vi "Collide_flappy.vi"(6 "Test":bool, 7 "obs_a?":bool, 8 "error in":errorcluster, 9 "Obs D_in":refnum<vi>[](array[refnum]), 10 "Obs U_in":refnum<vi>[](array[refnum]), 11 "ball in":refnum<vi>) -> (0 "error Out":errorcluster, 2 "bump":bool)   [LabVIEW 2014]
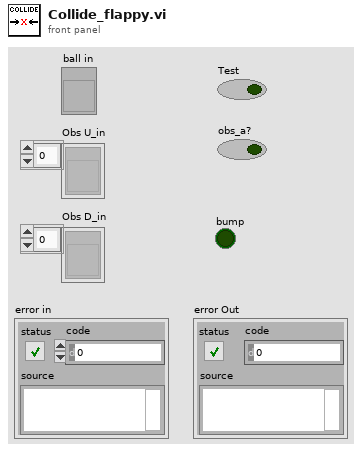
[diagram p1: front panel]
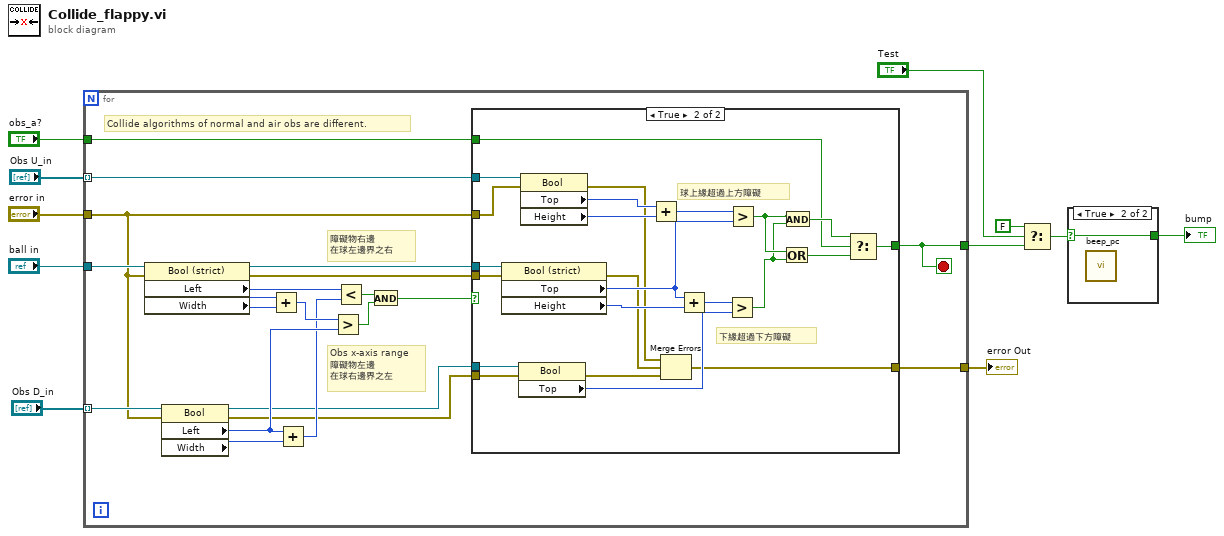
[diagram p0: block diagram]
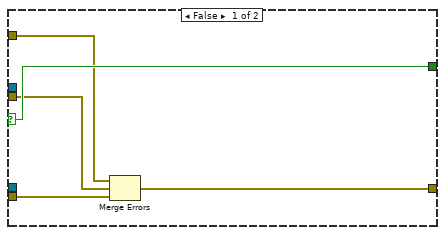
[diagram p3: hidden frame]
diagram:
  n1 = for {
    tunnel: "Obs U_in" -> [w22] mode=indexing
    tunnel: "ball in" -> [w21]
    tunnel: "Obs D_in" -> [w20] mode=indexing
    tunnel: "error in" -> [w15]
    tunnel: [w13] -> w3
    tunnel: [w14] -> w9
    tunnel: "obs_a?" -> [w12]
    stop <- w13 stop-if-true
    # "Collide algorithms of normal and air obs are different."
    # "障礙物右邊\n在球左邊界之右"
    # "Obs x-axis range\n障礙物左邊\n在球右邊界之左"
    n2 = property on="Property Node" class="Bool (strict)"(reference=w21, error in=w15) -> (reference out=w18:refnum<vi>, error out=w17:errorcluster, "Left"=w25:i32, "Width"=w26:u32)
    n3 = property on="Property Node" class="Bool"(reference=w20, error in=w15) -> (reference out=w19:refnum<vi>, error out=w16:errorcluster, "Left"=w28:i32, "Width"=w23:u32)
    n4 = Add(x=w25, y=w26) -> (x+y=w27:u32)
    n5 = Add(x=w28, y=w23) -> (x+y=w24:u32)
    n6 = Greater?(x=w27, y=w28) -> (0:w30:bool)
    n7 = Less?(x=w25, y=w24) -> (x < y?=w29:bool)
    n8 = And(x=w29, y=w30) -> (x .and. y?=w31:bool)
    n9 = case shown="True" w31 {
      selector: w31 -> [w36 _]
      tunnel: [w36 w41] -> w13
      tunnel: w22 -> [_ w54]
      tunnel: w18 -> [_ w53]
      tunnel: w19 -> [_ w52]
      tunnel: w17 -> [w33 w51]
      tunnel: w16 -> [w35 w50]
      tunnel: w15 -> [w32 w49]
      tunnel: [w34 w43] -> w14
      tunnel: w12 -> [_ w39]
      frame False {
        n10 = Merge Errors(w32, w33, w35) -> (w34:errorcluster)
      }
      frame True {
        # "球上緣超過上方障礙"
        # "下緣超過下方障礙"
        n11 = property on="Property Node" class="Bool (strict)"(reference=w53, error in=w51) -> (error out=w46:errorcluster, "Top"=w48:i32, "Height"=w57:u32)  [unwired: 1 out]
        n12 = property on="Property Node" class="Bool"(reference=w52, error in=w50) -> (error out=w45:errorcluster, "Top"=w55:i32)  [unwired: 1 out]
        n13 = property on="Property Node" class="Bool"(reference=w54, error in=w49) -> (error out=w44:errorcluster, "Top"=w58:i32, "Height"=w59:u32)  [unwired: 1 out]
        n14 = Add(x=w58, y=w59) -> (x+y=w47:u32)
        n15 = Merge Errors(w44, w46, w45) -> (w43:errorcluster)
        n16 = Add(x=w48, y=w57) -> (x+y=w56:u32)
        n17 = Greater?(x=w56, y=w55) -> (0:w37:bool)
        n18 = Greater?(x=w47, y=w48) -> (0:w38:bool)
        n19 = Or(x=w38, y=w37) -> (x .or. y?=w42:bool)
        n20 = And(x=w38, y=w37) -> (x .and. y?=w40:bool)
        n21 = Select(t=w40, s=w39, f=w42) -> (s? t:f=w41:bool)
      }
    }
  }
  "error Out" <- w9
  n22 = Select(t=FALSE, s="Test", f=w3) -> (s? t:f=w2:bool)
  n23 = case shown="True" w2 {
    selector: w2 -> [w60 w61]
    tunnel: [w60 w61] -> w1
    frame False {
    }
    frame True {
      n24 = call "beep_pc.vi"() -> ()  [unwired: 4 in, 1 out]
    }
  }
  "bump" <- w1
